vi "Create Frame Pattern Script.vi"(8 "error in (no error)":errorcluster, 9 "ChipID":u8, 10 "Frame_Data":T1={"Pattern_Name"="", "Operation Mode"=enum."Normal", "BurstLength"=enum."0", "FSN"=0, "Start_Addr"=0, "Data"=[], "R/W?"=enum."Read", "Opcode"=[], "ChipID"=1, "num of wait cycle of read"=0} {"Data" format="%x"; "Start_Addr" format="%x"}, 11 "BML_Frame_ReadCollect in":refnum<class "BML_Frame_ReadCollect.lvclass">) -> (0 "error out":errorcluster, 3 "BML_Frame_ReadCollect out":refnum<class "BML_Frame_ReadCollect.lvclass">)   [LabVIEW 2018, in "BML_Frame_ReadCollect.lvclass"]
uses:
  BML_Frame_ReadCollect.lvclass
  C:/P4 Workspace/PC Client/Solutions/5g_eap/HiSi/trunk/1.0/BML_Pattern_Gen_Refactor/Classes/BML_Frame_Root/BML_Frame_Root.lvclass
  Config_Read/Frame_Data.ctl
  Config_Read/OperationMode.ctl
  Config_Read/BurstLength.ctl
  Config_Read/RW_Option.ctl
  BML_Frame_Root/Special Frame.ctl
  BML_Frame_ReadCollect.lvclass/BML_Frame_ReadCollect.ctl
  BML_Frame_Root/BML_Frame_Root.lvclass/BML_Frame_Root.ctl
  BML_Frame_Cmd/BML_Frame_Command.lvclass
  BML_Frame_Addr/BML_Frame_Addr.lvclass
  Config_Read/Config_Read_BML.lvclass
  BML_Frame_Root/BML_Frame_Root.lvclass
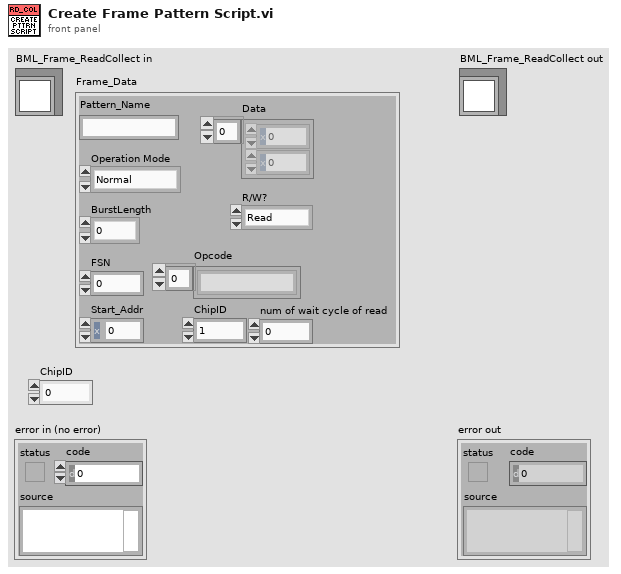
[diagram p1: front panel]
types:
  T1 = typedef "Config_Read_BML.lvclass/Frame_Data.ctl" = cluster{"Pattern_Name":string, "Operation Mode":T2, "BurstLength":T3, "FSN":u8, "Start_Addr":u16, "Data":u8[], "R/W?":T4, "Opcode":string[], "ChipID":u8, "num of wait cycle of read":i8}
  T2 = typedef "Config_Read_BML.lvclass/OperationMode.ctl" = enum8{"Normal", "ImmeEffect", "InitSlaveID", "LoadData"}
  T3 = typedef "Config_Read_BML.lvclass/BurstLength.ctl" = enum8{"0", "2", "3", "4", "5", "8", "16", "32"}
  T4 = typedef "Config_Read_BML.lvclass/RW_Option.ctl" = enum16{"Read", "Write", "R/W"}
  T5 = typedef "BML_Frame_Root.lvclass/Special Frame.ctl" = enum16{"Sync Header", "Protocol Header", "SW Trig", "SetID State", "Out SetID State", "SW Reset", "Wait", "SPI 4W FRM Start", "SPI 4W Wait", "SPI 4W FRM End", "SPI 4W Write Cmd", "SPI RD Collect Cmd", "SPI RD Value Cmd", "SPI 3W FRM Start", "SPI 3W Write Cmd", "SPI 3W FRM End", "SPI 3W Wait", "SPI 3W RD Cmd"}
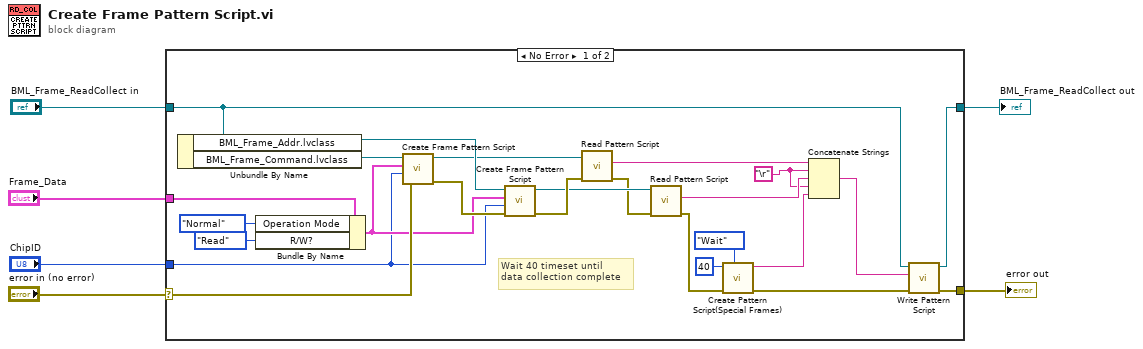
[diagram p0: block diagram]
diagram:
  n1 = case shown="No Error" "error in (no error)" {
    selector: "error in (no error)" -> [w28 w33]
    tunnel: [w9 w33] -> w5
    tunnel: [w8 w32] -> w4
    tunnel: "BML_Frame_ReadCollect in" -> [w11 w32]
    tunnel: "Frame_Data" -> [w30 _]
    tunnel: "ChipID" -> [w24 _]
    frame No Error {
      w14 = "\r"
      # "Wait 40 timeset until\ndata collection complete"
      n2 = Unbundle By Name(w11) -> ("BML_Frame_Addr.lvclass"=w27:refnum<class "BML_Frame_Addr.lvclass">, "BML_Frame_Command.lvclass"=w31:refnum<class "BML_Frame_Command.lvclass">)
      n3 = Bundle By Name(cluster=w30, "Operation Mode"=OperationMode."Normal", "R/W?"=RW_Option."Read") -> (w25:T1)
      n4 = call-dynamic "Create Frame Pattern Script.vi"("error in (no error)"=w28, "ChipID"=w24, "Frame_Data"=w25, "BML_Frame_Command in"=w31) -> ("error out"=w26:errorcluster, "BML_Frame_Command out"=w23:refnum<class "BML_Frame_Command.lvclass">)  [unwired: 6 in]
      n5 = call-dynamic "Create Frame Pattern Script.vi"("error in (no error)"=w26, "ChipID"=w24, "Frame_Data"=w25, "BML_Frame_Addr in"=w27) -> ("error out"=w22:errorcluster, "BML_Frame_Addr out"=w21:refnum<class "BML_Frame_Addr.lvclass">)  [unwired: 6 in]
      n6 = call "Read Pattern Script.vi"("error in (no error)"=w22, "BML_Frame_Root in"=w23) -> ("error out"=w20:errorcluster, "Pattern Script"=w16:string)  [unwired: 7 in, 1 out]
      n7 = call "Read Pattern Script.vi"("error in (no error)"=w20, "BML_Frame_Root in"=w21) -> ("error out"=w19:errorcluster, "Pattern Script"=w15:string)  [unwired: 7 in, 1 out]
      n8 = call "Create Pattern Script(Special Frames).vi"("Special Frame Type"=Special_Frame."Wait", "error in (no error)"=w19, "Num of Timeset"=u32 40) -> ("error out"=w10:errorcluster, "string out"=w13:string)  [unwired: 7 in]
      n9 = Concatenate Strings(w16, w14, w15, w14, w13) -> (w12:string)
      n10 = call "Write Pattern Script.vi"("error in (no error)"=w10, "Pattern Script"=w12, "BML_Frame_Root in"=w11) -> ("error out"=w9:errorcluster, "BML_Frame_Root out"=w8:refnum<class "BML_Frame_ReadCollect.lvclass">)  [unwired: 7 in]
    }
    frame Error {
    }
  }
  "error out" <- w5
  "BML_Frame_ReadCollect out" <- w4
